vi "Create Default Instrument Addon.vi"(8 "Error In":errorcluster, 11 "Target In":refnum<k24>) -> (0 "Error Out":errorcluster, 2 "Instrument Addon Refnum":T1=18446744073709551615 format="%.0x", 3 "Target Out":refnum<k24>)   [LabVIEW 2020, in "Instrument Addon Scripting API.lvlib"]
uses:
  Instrument Addon Scripting API.lvlib
  NationalInstruments.VeriStand.SystemDefinitionAPI
  <vilib>/NI VeriStand/Custom Device API/Custom Device Item Ref.ctl
  Shared Directory/Constants.vi
  Shared Directory/Instrument Addon Shared.lvlib
  <vilib>/NI VeriStand/Custom Device Tools/Custom Device Utility Library/Custom Device Utility Library.lvlib
  <vilib>/NI VeriStand/Custom Device API/Custom Device API.lvlib
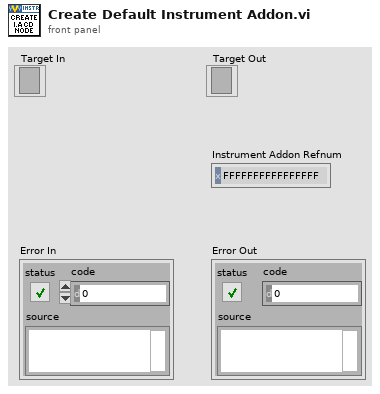
[diagram p1: front panel]
types:
  T1 = typedef "Custom Device API.lvlib/Custom Device Item Ref.ctl" = u64
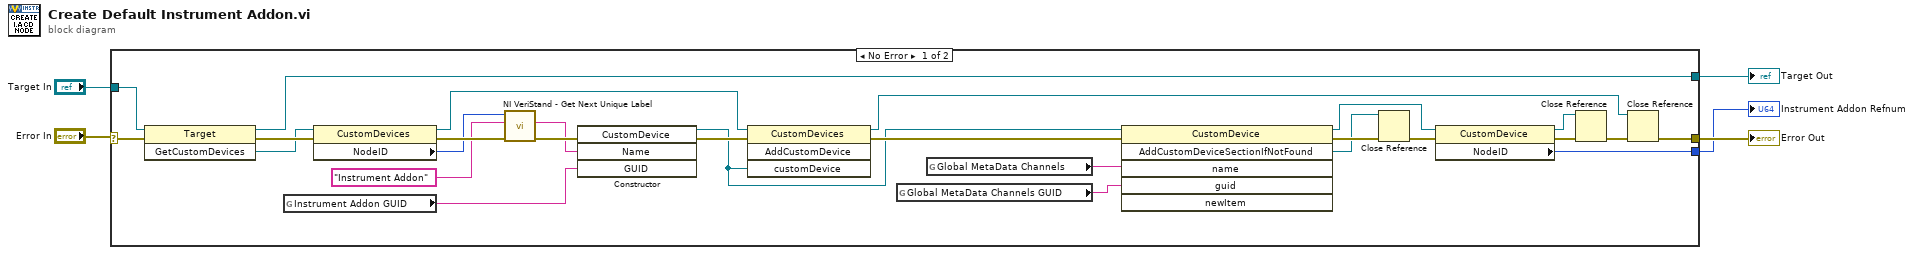
[diagram p0: block diagram]
diagram:
  n1 = case shown="No Error" "Error In" {
    selector: "Error In" -> [w20 w34]
    tunnel: [w32 _] -> w1
    tunnel: "Target In" -> [w31 w33]
    tunnel: [w18 w34] -> w3
    tunnel: [w16 w33] -> w2
    frame No Error {
      n2 = invoke class="Target" method="GetCustomDevices"(reference=w31, error in=w20) -> (reference out=w16:refnum<k24>, error out=w24:errorcluster, "GetCustomDevices"=w23:refnum<k24>)  [unwired: 1 in]
      n3 = global read "Constants.vi" "Instrument Addon GUID"() -> (w22:string)
      n4 = property class="CustomDevices"(reference=w23, error in=w24) -> (reference out=w27:refnum<k24>, error out=w29:errorcluster, "NodeID"=w25:u64)
      n5 = call <vilib>:"NI VeriStand - Get Next Unique Label.vi"("error in (no error)"=w29, "Label"="Instrument Addon" ("Name"), "Parent Ref in"=w25) -> ("error out"=w30:errorcluster, "Label out"=w28:string)  [unwired: 5 in, 2 out]
      n6 = constructor class="CustomDevice"(error in=w30, "Name"=w28, "GUID"=w22) -> (reference out=w12:refnum<k24>, error out=w21:errorcluster)  [unwired: 2 in, 3 out]
      n7 = invoke class="CustomDevices" method="AddCustomDevice"(reference=w27, error in=w21, "customDevice"=w12) -> (reference out=w17:refnum<k24>, error out=w13:errorcluster)  [unwired: 1 in, 2 out]
      n8 = global read "Constants.vi" "Global MetaData Channels GUID"() -> (w11:string)
      n9 = global read "Constants.vi" "Global MetaData Channels"() -> (w6:string)
      n10 = invoke class="CustomDevice" method="AddCustomDeviceSectionIfNotFound"(reference=w12, error in=w13, "name"=w6, "guid"=w11) -> (reference out=w8:refnum<k24>, error out=w10:errorcluster, "AddCustomDeviceSectionIfNotFound"=w9:refnum<k24>)  [unwired: 2 in, 3 out]
      n11 = Close Reference(reference=w9, error in (no error)=w10) -> (error out=w7:errorcluster)
      n12 = property class="CustomDevice"(reference=w8, error in=w7) -> (reference out=w14:refnum<k24>, error out=w15:errorcluster, "NodeID"=w32:u64)
      n13 = Close Reference(reference=w14, error in (no error)=w15) -> (error out=w19:errorcluster)
      n14 = Close Reference(reference=w17, error in (no error)=w19) -> (error out=w18:errorcluster)
    }
    frame Error {
    }
  }
  "Error Out" <- w3
  "Target Out" <- w2
  "Instrument Addon Refnum" <- w1
